vi "Create and Read PWM Output.vi"(8 "error in":errorcluster, 10 "channel settings in":T1[](array[typedef]), 11 "NI 9475 Test in":refnum<class "NI 9475 Test.lvclass">) -> (0 "error out":errorcluster, 2 "channel settings out":T1[](array[typedef]), 3 "NI 9475 Test out":refnum<class "NI 9475 Test.lvclass">)   [LabVIEW 2017, in "NI 9475 Test.lvclass"]
uses:
  NI 9475 Test.lvclass
  Scripting/Modules/Mode Classes/Controls/pwm channel settings.ctl
  Scripting/Modules/Channel Classes/PWM Output Channel/Frequency.ctl
  Scripting/Modules/NI 9475/NI 9475.lvclass
  Scripting/Modules/Channel Classes/PWM Output Channel/PWM Output Channel.lvclass
  Scripting/Scan Engine Scripting.lvlib
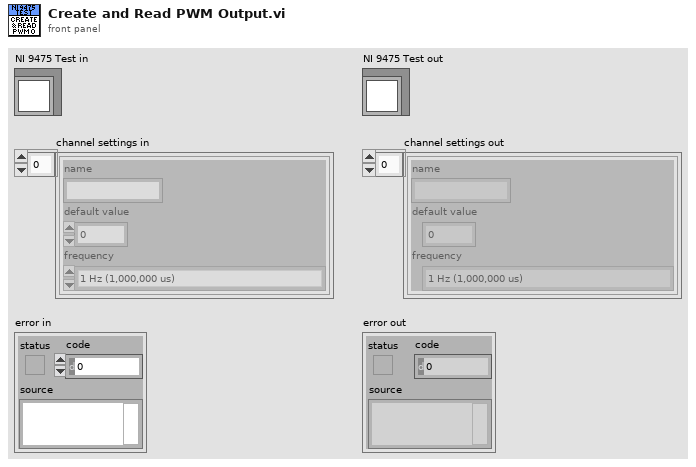
[diagram p1: front panel]
types:
  T1 = typedef "Scan Engine Scripting.lvlib/pwm channel settings.ctl" = cluster{"name":string, "default value":dbl, "frequency":T2}
  T2 = typedef "Scan Engine Scripting.lvlib/PWM Output Channel.lvclass/Frequency.ctl" = enum16{"1 Hz (1,000,000 us)", "50 Hz (20,000 us)", "250 Hz (4,000 us)", "500 Hz (2,000 us)", "1 kHz (1,000 us)", "5 kHz (200 us)", "10 kHz (100 us)", "20 kHz (50 us)"}
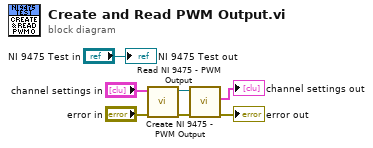
[diagram p0: block diagram]
diagram:
  n1 = call "Create NI 9475 - PWM Output.vi"("error in"="error in", "channel settings"="channel settings in") -> ("error out"=w7:errorcluster, "NI 9475 out"=w5:refnum<class "NI 9475.lvclass">)  [unwired: 8 in]
  n2 = call "Read NI 9475 - PWM Output.vi"("error in (no error)"=w7, "NI 9475 in"=w5) -> ("error out"=→"error out":errorcluster, "channel settings"=→"channel settings out":T1[])  [unwired: 7 in, 1 out]
  "NI 9475 Test out" <- "NI 9475 Test in"
